vi "例5.16  波形数组.vi"() -> ()   [LabVIEW 2017]
uses:
  <vilib>/measure/NI_MABase.lvlib
panel:
  out "dt1":dbl
  out "Y1":dbl[](array[numeric])
  in  "phase":dbl caption="相位" format="%.2p"
  in  "amplitude":dbl=1.0 caption="幅值" format="%0.2p"
  in  "frequency":dbl=10.0 caption="频率" format="%0.2p"
  in  "sampling info":cluster{"Fs":dbl, "#s":dbl}={"Fs"=1000.0, "#s"=1000.0} caption="采样信息" {"Fs" format="%.2p"}
  out "生成的波形":waveform(dbl)[](graph)
  in  "采样信息":cluster{"Fs":dbl, "#s":dbl}={"Fs"=1000.0, "#s"=1000.0} {"Fs" format="%.2p"}
  in  "相位":dbl format="%.2p"
  in  "幅值":dbl=1.0 format="%0.2p"
  in  "频率":dbl=10.0 format="%0.2p"
  out "dt0":dbl
  out "Y0":dbl[](array[numeric])
  # "正弦波 参数"
  # "方波 参数"
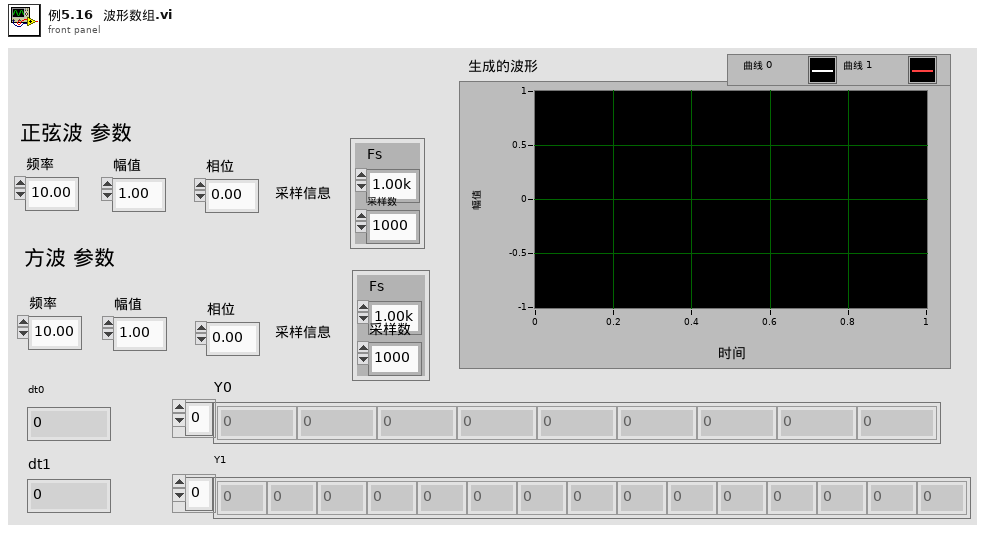
[diagram p1: front panel]
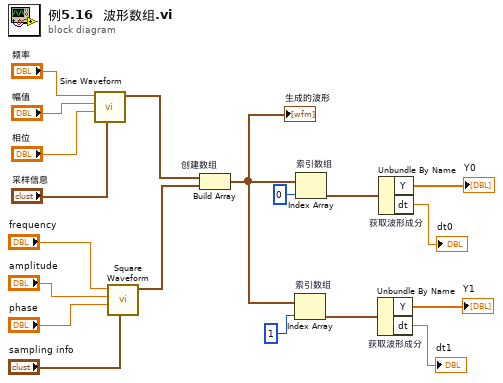
[diagram p0: block diagram]
diagram:
  n1 = call <vilib>:"Sine Waveform.vi"("sampling info"="采样信息", "phase"="相位", "amplitude"="幅值", "frequency"="频率") -> ("signal out"=w9:waveform(dbl))  [unwired: 6 in, 1 out]
  n2 = call <vilib>:"Square Waveform.vi"("sampling info"="sampling info", "phase"="phase", "amplitude"="amplitude", "frequency"="frequency") -> ("signal out"=w8:waveform(dbl))  [unwired: 6 in, 1 out]
  n3 = Build Array "创建数组"(w9, w8) -> (w1:waveform(dbl)[])
  "生成的波形" <- w1
  n4 = Index Array "索引数组"(array=w1, index=1 ("索引")) -> (element=w3:waveform(dbl))
  n5 = Index Array "索引数组"(array=w1, index=0 ("索引")) -> (element=w6:waveform(dbl))
  n6 = Unbundle By Name "获取波形成分"(w3) -> ("Y"=→"Y1":dbl[], "dt"=→"dt1":dbl)
  n7 = Unbundle By Name "获取波形成分"(w6) -> ("Y"=→"Y0":dbl[], "dt"=→"dt0":dbl)
